vi "Result.vi"(8 "error in (no error)":errorcluster, 10 "Result":T1={"Name"="", "Description"="", "Status"=enum."Passed", "Result Type"=enum."Test Suite", "Execution Time"=0.0, "Data"={"Expected"=variant, "Actual"=variant, "Delta"=variant}}, 11 "Icon Decorator In":refnum<class "Icon Decorator.lvclass">) -> (0 "error out":errorcluster)   [LabVIEW 2020, in "Icon Decorator.lvclass"]
uses:
  Icon Decorator.lvclass
  Core/Result/Result.ctl
  Core/Result/Status.ctl
  Core/Result/Type.ctl
  Core/Result/Result.lvlib
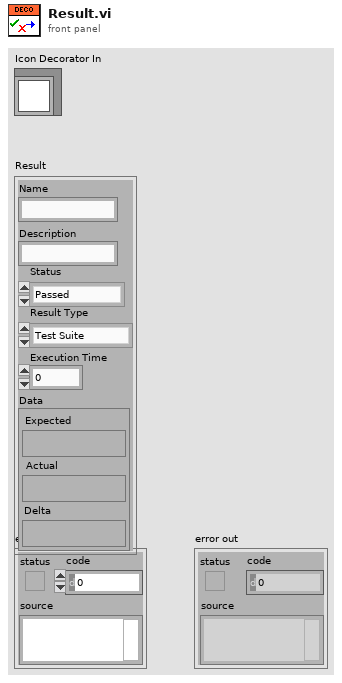
[diagram p1: front panel]
types:
  T1 = typedef "Result.lvlib/Result.ctl" = cluster{"Name":string, "Description":string, "Status":T2, "Result Type":T3, "Execution Time":dbl, "Data":cluster{"Expected":variant, "Actual":variant, "Delta":variant}}
  T2 = typedef "Result.lvlib/Status.ctl" = enum16{"", "Passed", "Failed", "Error", "Skipped", "Setup Error", "Broken", "Teardown Error"}
  T3 = typedef "Result.lvlib/Type.ctl" = enum16{"Test Case", "Test Suite", "Test Run", "Pass", "Fail", "Skip", "Pass if", "Fail if", "Pass if Error", "Fail if Error", "Pass if Equal", "Fail if Equal"}
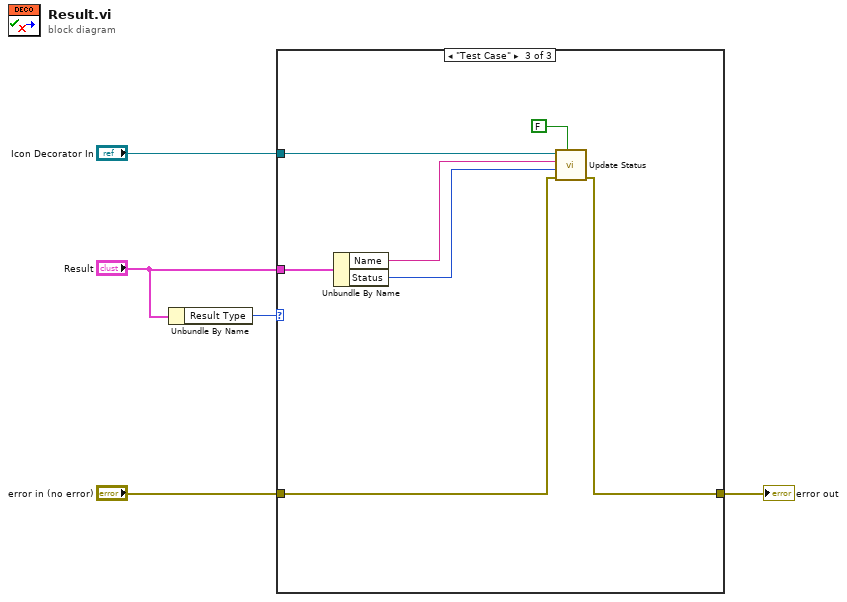
[diagram p0: block diagram]
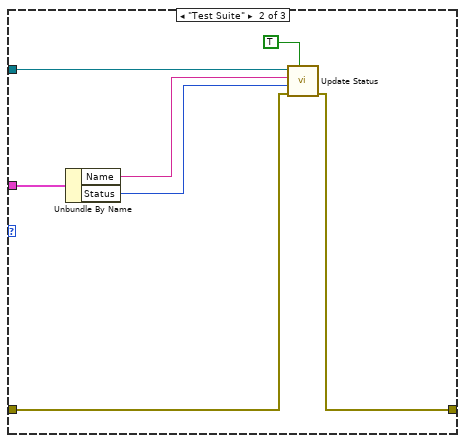
[diagram p3: hidden frame]
diagram:
  n1 = Unbundle By Name("Result") -> ("Result Type"=w5:T3)
  n2 = case shown="\"Test Case\"" w5 {
    tunnel: "Icon Decorator In" -> [_ w11 w18]
    tunnel: "error in (no error)" -> [w6 w9 w16]
    tunnel: "Result" -> [_ w13 w20]
    tunnel: [w6 w8 w15] -> w1
    frame Default {
    }
    frame "Test Suite" {
      n3 = Unbundle By Name(w13) -> ("Name"=w12:string, "Status"=w10:T2)
      n4 = call "Update Status.vi"("Check overlay?"=TRUE, "error in (no error)"=w9, "Status"=w10, "Case"=w12, "Icon Decorator In"=w11) -> ("error out"=w8:errorcluster)  [unwired: 6 in]
    }
    frame "Test Case" {
      n5 = Unbundle By Name(w20) -> ("Name"=w19:string, "Status"=w17:T2)
      n6 = call "Update Status.vi"("Check overlay?"=FALSE, "error in (no error)"=w16, "Status"=w17, "Case"=w19, "Icon Decorator In"=w18) -> ("error out"=w15:errorcluster)  [unwired: 6 in]
    }
  }
  "error out" <- w1
